vi "Facade.vi"(0 "Data In":T8, 2 "Display State In":T2={"Nspeakers"=0, "actions"=[], "Wspeaker"=13, "hover"={"type"=enum."None", "index"=0}, "locked"=FALSE, "states"=[], "sel speak"=13, "selected"=refnum, "Events"={"Selection change"=refnum}}, 3 "Container State":T7) -> (6 "Data Out":T8, 7 "Display State Out":T2={"Nspeakers"=0, "actions"=[], "Wspeaker"=13, "hover"={"type"=enum."None", "index"=0}, "locked"=FALSE, "states"=[], "sel speak"=13, "selected"=refnum, "Events"={"Selection change"=refnum}}, 8 "Action":T1)   [LabVIEW 2015, in "SAC Config.xctl"]
uses:
  SAC Config.xctl
  <vilib>/_xctls/Action.ctl
  <vilib>/_xctls/XControlSupport.lvlib
  Speaker State.ctl
  Hover Item.ctl
  <vilib>/_xctls/Container State.ctl
  Data.vi
  State.vi
  Hover Data.ctl
  Events.ctl
  Selection changed.ctl
panel:
  out "angle":string
  out "selected":picture
  out "speakers":picture
  out "back":picture
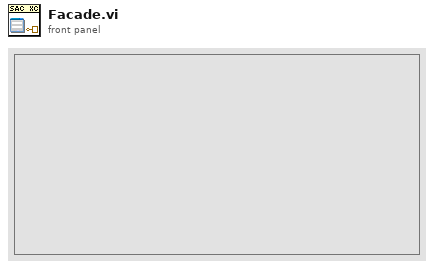
[diagram p1: front panel]
types:
  T1 = typedef "XControlSupport.lvlib/Action.ctl" = cluster{"Data Changed?":bool, "State Changed?":bool, "Action Name":string}
  T2 = typedef "SAC Config.xctl/State.vi" = cluster{"Nspeakers":i32, "actions":string[], "Wspeaker":i32, "hover":T3, "locked":bool, "states":T5[], "sel speak":i32, "selected":refnum<vi>, "Events":T6}
  T3 = typedef "SAC Config.xctl/Hover Data.ctl" = cluster{"type":T4, "index":i32}
  T4 = typedef "SAC Config.xctl/Hover Item.ctl" = enum16{"None", "Speaker"}
  T5 = typedef "SAC Config.xctl/Speaker State.ctl" = cluster{"cal":bool, "selected":bool}
  T6 = typedef "SAC Config.xctl/Events.ctl" = cluster{"Selection change":refnum<user-event>}
  T7 = typedef "XControlSupport.lvlib/Container State.ctl" = cluster{"Indicator?":bool, "Run Mode?":bool, " Refnum":refnum<vi>}
  T8 = typedef "SAC Config.xctl/Data.vi" = i32
  T9 = typedef "LVPoint32TypeDef.ctl" = cluster{"Horizontal":i32, "Vertical":i32}
  T10 = cluster{"Min Control Width":i32, "Min Control Height":i32}
  T11 = typedef "LVPointTypeDef.ctl" = cluster{"Horizontal":i16, "Vertical":i16}
  T12 = typedef "SAC Config.xctl/Layout.ctl" = cluster{"origin":cluster{"X":i32, "Y":i32}, "Items":T13[], "ring diameter":i32}
  T13 = typedef "SAC Config.xctl/Item.ctl" = cluster{"center":cluster{"X":i32, "Y":i32}, "angle":dbl}
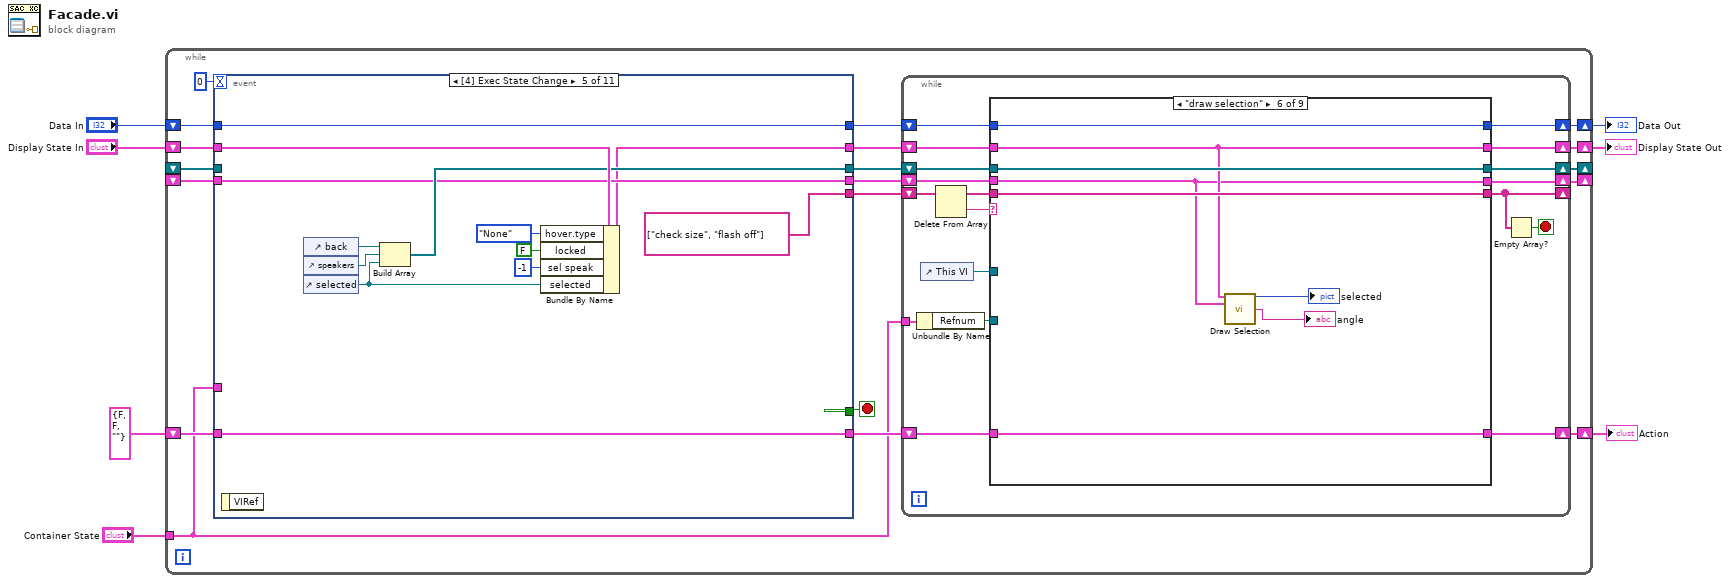
[diagram p0: block diagram]
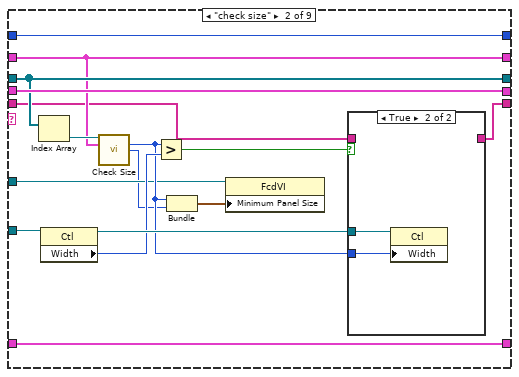
[diagram p3: hidden frame]
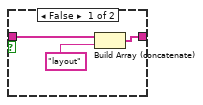
[diagram p4: hidden frame]
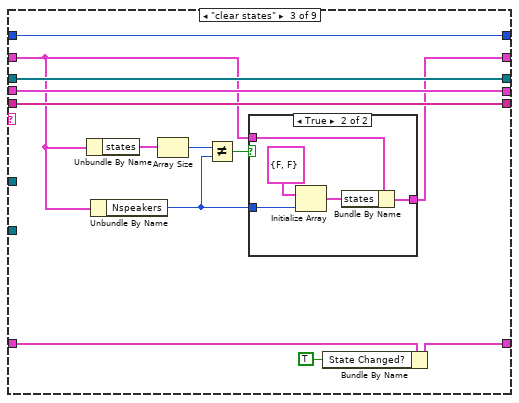
[diagram p5: hidden frame]
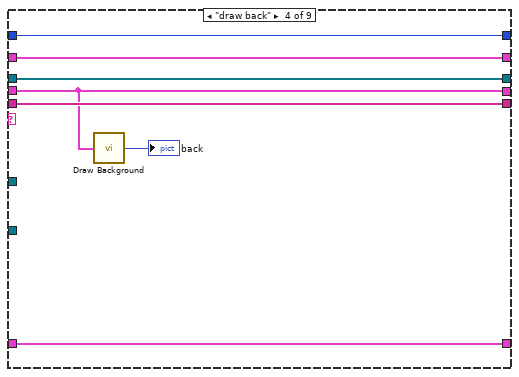
[diagram p7: hidden frame]
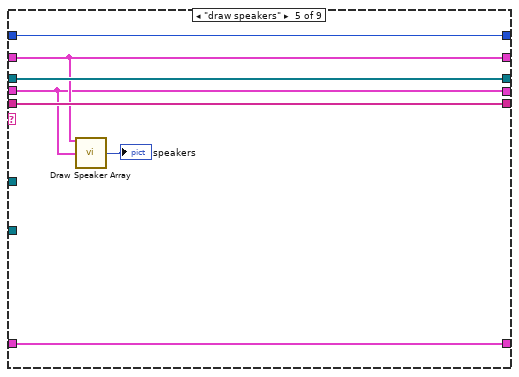
[diagram p8: hidden frame]
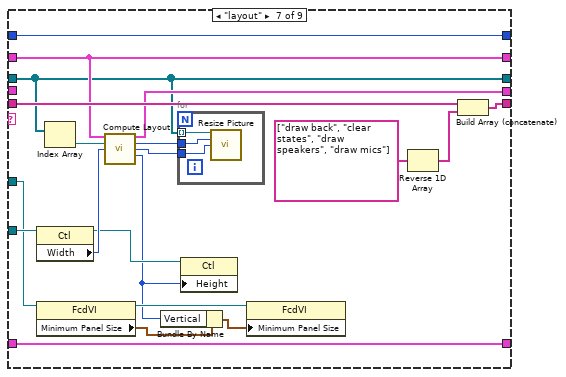
[diagram p9: hidden frame]
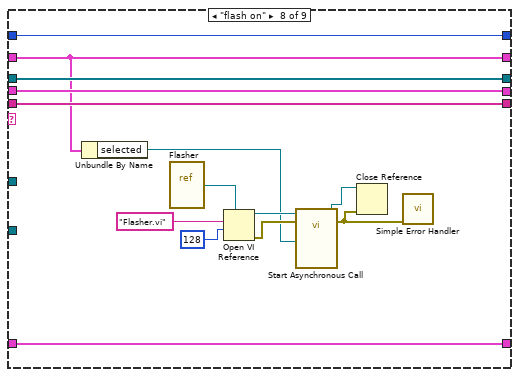
[diagram p10: hidden frame]
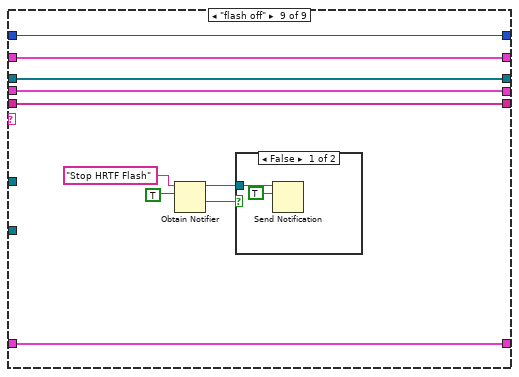
[diagram p11: hidden frame]
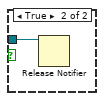
[diagram p12: hidden frame]
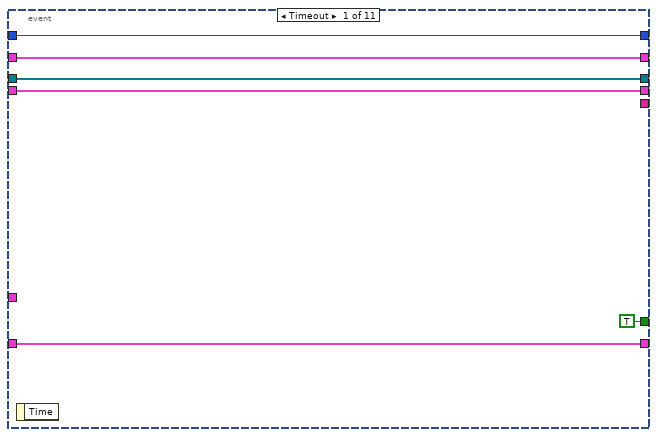
[diagram p13: hidden frame]
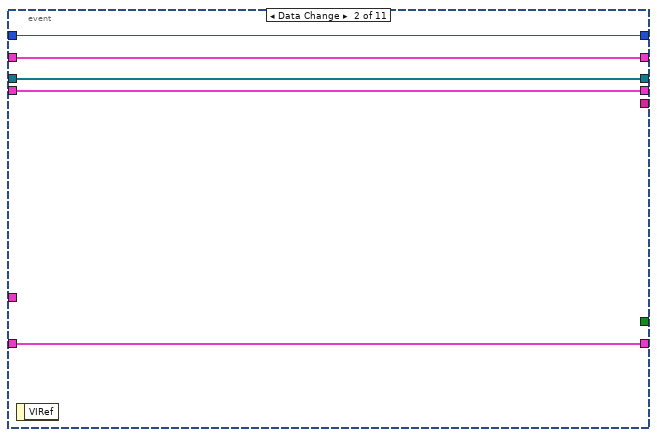
[diagram p14: hidden frame]
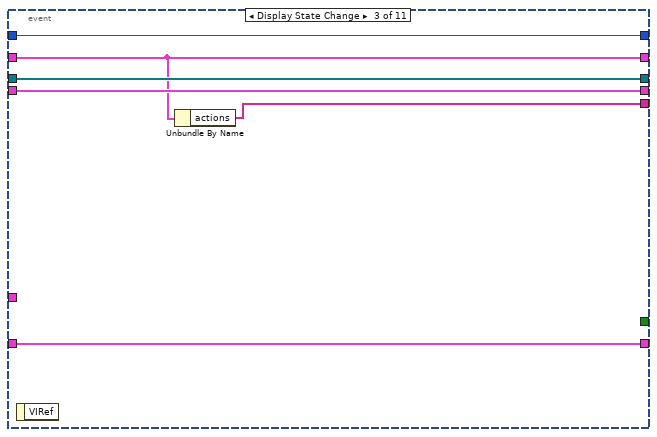
[diagram p15: hidden frame]
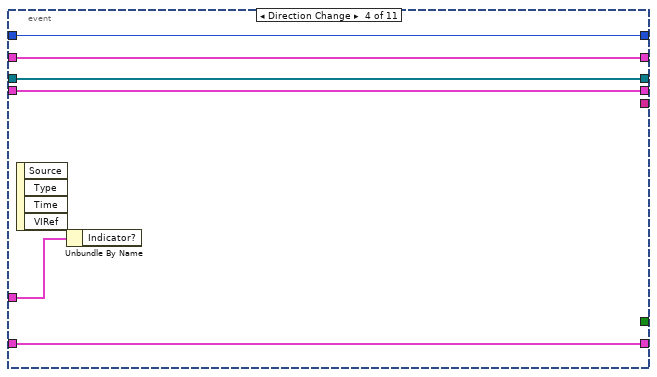
[diagram p16: hidden frame]
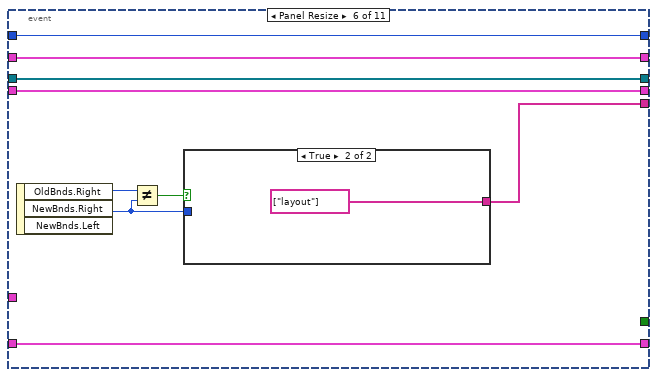
[diagram p17: hidden frame]
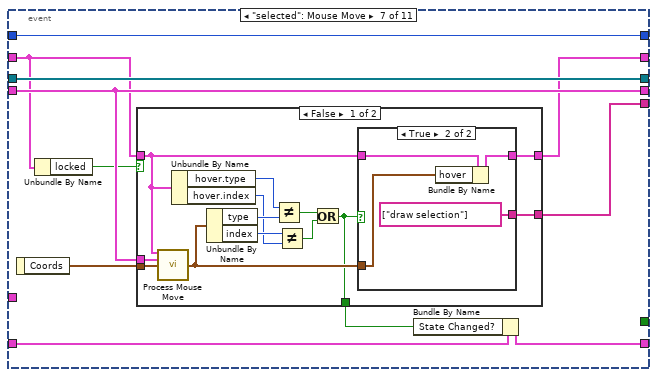
[diagram p19: hidden frame]
diagram:
  n1 = while {
    shift-right: [w15] -> w4
    shift-left: "Display State In" -> [w26]
    tunnel: "Container State" -> [w11]
    shift-right: [w16] -> w7
    shift-left: "Data In" -> [w23]
    shift-right: [w13] -> w2
    shift-left: T1 {"Data Changed?"=FALSE, "State Changed?"=FALSE, "Action Name"=""} ("Action") -> [w22]
    shift-right: [w14] -> _
    shift-left: _ -> [w21]
    shift-right: [w10] -> _
    shift-left: _ -> [w9]
    stop <- w25 stop-if-true
    n2 = event shown="[4] Exec State Change" {
      selector: _ -> [_ _ _ _ _ _ _ _ _ _ _]
      dyn-events: _ -> [_ _ _ _ _ _ _ _ _ _ _]
      timeout: 0 -> [_ _ _ _ _ _ _ _ _ _ _]
      tunnel: w26 -> [w166 w172 w174 w184 w194 w207 w210 w246 w286 w299 w305]
      tunnel: [w166 w172 w174 w184 w190 w207 w214 w245 w285 w299 w310] -> w18
      tunnel: [TRUE _ _ _ _ _ _ _ _ _ _] -> w25
      tunnel: w11 -> [_ _ _ w185 _ _ _ _ _ _ _]
      tunnel: w23 -> [w165 w173 w179 w183 w198 w206 w219 w252 w290 w303 w318]
      tunnel: [w165 w173 w179 w183 w198 w206 w219 w252 w290 w303 w318] -> w17
      tunnel: [w167 w171 w178 w182 w197 w205 w213 w244 w284 w302 w313] -> w12
      tunnel: w22 -> [w167 w171 w178 w182 w197 w205 w218 w251 w289 w302 w317]
      tunnel: [w164 w170 w177 w181 w193 w204 w217 w250 w288 w301 w316] -> w19
      tunnel: w21 -> [w164 w170 w177 w181 _ w204 w217 w250 w288 w301 w316]
      tunnel: [_ _ w175 _ string[] ["check size", "flash off"] w199 w211 w242 w282 _ string[] ["draw selection", "draw speakers"] ("String")] -> w20
      tunnel: w9 -> [w163 w169 w176 w180 w191 w200 w215 w248 w287 w300 w315]
      tunnel: [w163 w169 w176 w180 w191 w200 w215 w248 w287 w300 w315] -> w8
      event Timeout {
        n3 = event-data() -> ()  [unwired: 1 in, 1 out]
      }
      event Data Change {
        n4 = event-data() -> ()  [unwired: 1 in, 1 out]
      }
      event Display State Change {
        n5 = event-data() -> ()  [unwired: 1 in, 1 out]
        n6 = Unbundle By Name(w174) -> ("actions"=w175:string[])
      }
      event Direction Change {
        n7 = event-data() -> ()  [unwired: 1 in, 4 out]
        n8 = Unbundle By Name(w185) -> ()  [unwired: 1 out]
      }
      event Exec State Change {
        n9 = event-data() -> ()  [unwired: 1 in, 1 out]
        n10 = control-ref of="back"() -> (w195:refnum<vi>)
        n11 = control-ref of="speakers"() -> (w196:refnum<vi>)
        n12 = control-ref of="selected"() -> (w186:refnum<vi>)
        n13 = Build Array(w195, w196, w186) -> (w193:refnum<vi>[])
        n14 = Bundle By Name(cluster=w194, "hover.type"=Hover_Item."None", "locked"=FALSE, "sel speak"=-1, "selected"=w186) -> (w190:T2)
      }
      event Panel Resize {
        n15 = event-data() -> ("OldBnds.Right"=w203:i16, "NewBnds.Right"=w202:i16)  [unwired: 1 in, 1 out]
        n16 = Not Equal?(x=w203, y=w202) -> (x != y?=w201:bool)
        n17 = case shown="True" w201 {
          tunnel: w202 -> [_ _]
          tunnel: [_ string[] ["layout"] ("String")] -> w199
          frame False {
          }
          frame True {
          }
        }
      }
      event "selected": Mouse Move {
        n18 = event-data() -> ("Coords"=w216:T9)  [unwired: 1 in]
        n19 = Unbundle By Name(w210) -> ("locked"=w209:bool)
        n20 = case shown="False" w209 {
          tunnel: w216 -> [w232 _]
          tunnel: w215 -> [w231 _]
          tunnel: [w223 w238] -> w214
          tunnel: [w222 _] -> w212
          tunnel: [w221 _] -> w211
          tunnel: w210 -> [w220 w238]
          frame False {
            n21 = call "Process Mouse Move.vi"("State"=w220, "Layout"=w231, "Coords"=w232) -> ("Hover Data"=w224:T3)  [unwired: 12 in]
            n22 = Unbundle By Name(w220) -> ("hover.type"=w229:T4, "hover.index"=w226:i32)
            n23 = Unbundle By Name(w224) -> ("type"=w230:T4, "index"=w227:i32)
            n24 = Not Equal?(x=w229, y=w230) -> (x != y?=w228:bool)
            n25 = Not Equal?(x=w227, y=w226) -> (x != y?=w225:bool)
            n26 = Or(x=w228, y=w225) -> (x .or. y?=w222:bool)
            n27 = case shown="True" w222 {
              tunnel: w224 -> [_ w235]
              tunnel: w220 -> [w233 w237]
              tunnel: [w233 w236] -> w223
              tunnel: [_ string[] ["draw selection"] ("String")] -> w221
              frame False {
              }
              frame True {
                n28 = Bundle By Name(cluster=w237, "hover"=w235) -> (w236:T2)
              }
            }
          }
          frame True {
          }
        }
        n29 = Bundle By Name(cluster=w218, "State Changed?"=w212) -> (w213:T1)
      }
      event "selected": Mouse Down {
        n30 = event-data() -> ("PlatMods.Shift"=w239:bool)  [unwired: 1 in]
        n31 = Unbundle By Name(w246) -> ("hover.type"=w249:T4, "hover.index"=w247:i32, "sel speak"=w240:i32, "locked"=w241:bool)
        n32 = case shown="False" w241 {
          tunnel: w249 -> [w260 _]
          tunnel: w247 -> [w259 _]
          tunnel: w246 -> [w258 w280]
          tunnel: [w257 w280] -> w245
          tunnel: [w256 _] -> w243
          tunnel: [w255 _] -> w242
          tunnel: w240 -> [w254 _]
          tunnel: w239 -> [w253 _]
          frame False {
            n33 = case shown="\"Speaker\"" w260 {
              tunnel: w258 -> [w264 w267]
              tunnel: w259 -> [_ w270]
              tunnel: [w262 w274] -> w257
              tunnel: [TRUE TRUE] -> w256
              tunnel: [_ string[] ["draw selection", "draw speakers"] ("String")] -> w255
              tunnel: w254 -> [_ w273]
              tunnel: w253 -> [_ w272]
              frame "None", Default {
                n34 = Bundle By Name(cluster=w264, "sel speak"=-1) -> (w262:T2)
              }
              frame "Speaker" {
                n35 = Unbundle By Name(w267) -> ("Events.Selection change"=w269:refnum<user-event>)
                n36 = Unbundle By Name(w267) -> ("states"=w276:T5[])
                n37 = call "Update Speaker Selection.vi"("states in"=w276, "index"=w270, "sel speak"=w273, "Shift"=w272) -> ("states out"=w266:T5[])  [unwired: 11 in]
                n38 = Bundle By Name(cluster=w267, "states"=w266, "sel speak"=w270) -> (w274:T2)
                n39 = for {
                  tunnel: w266 -> [w279] mode=indexing
                  tunnel: [w277] -> w265 mode=indexing if=w278
                  i -> [w277]
                  n40 = Unbundle By Name(w279) -> ("selected"=w278:bool)
                }
                n41 = Bundle(w265) -> (w268:cluster{i32[]})  [unwired: 1 in]
                n42 = Generate User Event(user event=w269, event data cluster=w268) -> ()  [unwired: 2 in, 2 out]
              }
            }
          }
          frame True {
          }
        }
        n43 = Bundle By Name(cluster=w251, "State Changed?"=w243) -> (w244:T1)
      }
      event Mouse Leave {
        n44 = event-data() -> ()  [unwired: 1 in, 1 out]
        n45 = Unbundle By Name(w286) -> ("locked"=w281:bool)
        n46 = case shown="False" w281 {
          tunnel: w286 -> [w296 w297]
          tunnel: [w295 w297] -> w285
          tunnel: [TRUE _] -> w283
          tunnel: [string[] ["draw selection"] ("String") _] -> w282
          frame False {
            n47 = Bundle By Name(cluster=w296, "sel speak"=-1, "hover.type"=Hover_Item."None") -> (w295:T2)
          }
          frame True {
          }
        }
        n48 = Bundle By Name(cluster=w289, "State Changed?"=w283) -> (w284:T1)
      }
      event "selected": Shortcut Menu Activation? {
        n49 = event-data() -> ()  [unwired: 1 in, 1 out]
        n50 = Unbundle By Name(w299) -> ("locked"=w298:bool)
        n51 = event-data("Discard?"=w298) -> ()  [unwired: 1 in, 1 out]
      }
      event "selected": Shortcut Menu Selection (User) {
        n52 = event-data() -> ("ItemTag"=w311:string)  [unwired: 1 in]
        n53 = Unbundle By Name(w305) -> ("states"=w314:T5[])
        n54 = for {
          tunnel: w314 -> [w323] mode=indexing
          tunnel: w311 -> [w325]
          tunnel: [w324] -> w309 mode=indexing
          tunnel: [w321] -> w306 mode=indexing if=w320
          i -> [w321]
          n55 = Unbundle By Name(w323) -> ("selected"=w322:bool)
          n56 = Unbundle By Name(w323) -> ("cal"=w319:bool)
          n57 = case shown="\"cmClearAll\"" w325 {
            tunnel: w319 -> [_ _ w329 _ w334]
            tunnel: [FALSE TRUE w328 FALSE w331] -> w320
            tunnel: w322 -> [_ _ _ _ w332]
            frame "False", Default {
            }
            frame "cmSelectAll" {
            }
            frame "cmSelectIncomplete" {
              n58 = Not(x=w329) -> (.not. x?=w328:bool)
            }
            frame "cmClearAll" {
            }
            frame "cmClearComplete" {
              n59 = Not(x=w334) -> (.not. x?=w333:bool)
              n60 = And(x=w333, y=w332) -> (x .and. y?=w331:bool)
            }
          }
          n61 = Bundle By Name(cluster=w323, "selected"=w320) -> (w324:T5)
        }
        n62 = Unbundle By Name(w305) -> ("Events.Selection change"=w304:refnum<user-event>)
        n63 = Bundle By Name(cluster=w317, "State Changed?"=TRUE) -> (w313:T1)
        n64 = Bundle By Name(cluster=w305, "states"=w309) -> (w310:T2)
        n65 = Bundle(w306) -> (w307:cluster{i32[]})  [unwired: 1 in]
        n66 = Generate User Event(user event=w304, event data cluster=w307) -> ()  [unwired: 2 in, 2 out]
      }
    }
    n67 = while {
      shift-right: [w39] -> w16
      shift-left: w17 -> [w43]
      shift-right: [w38] -> w15
      shift-left: w18 -> [w42]
      shift-right: [w37] -> w14
      shift-left: w19 -> [w41]
      shift-right: [w35] -> w13
      shift-left: w12 -> [w40]
      shift-right: [w36] -> _
      shift-left: w20 -> [w34]
      tunnel: w11 -> [w28]
      shift-right: [w30] -> w10
      shift-left: w8 -> [w29]
      stop <- w44 stop-if-true
      n68 = Unbundle By Name(w28) -> ("Refnum"=w27:refnum<vi>)
      n69 = control-ref of="This VI"() -> (w31:refnum<vi>)
      n70 = Delete From Array(array=w34) -> (deleted portion=w32:string, array with subset deleted=w33:string[])  [unwired: 2 in]
      n71 = case shown="\"draw selection\"" w32 {
        tunnel: w43 -> [w50 w66 w84 w97 w104 w112 w132 w149 w159]
        tunnel: w42 -> [w49 w61 w76 w96 w100 w108 w129 w144 w158]
        tunnel: w41 -> [w48 w63 w83 w95 w103 w111 w122 w148 w157]
        tunnel: w33 -> [w47 w56 w82 w94 w102 w110 w131 w147 w156]
        tunnel: w40 -> [w46 w65 w81 w93 w101 w109 w130 w146 w155]
        tunnel: [w50 w66 w84 w97 w104 w112 w132 w149 w159] -> w39
        tunnel: [w49 w61 w79 w96 w100 w108 w129 w144 w158] -> w38
        tunnel: [w48 w63 w83 w95 w103 w111 w122 w148 w157] -> w37
        tunnel: [w47 w55 w82 w94 w102 w110 w127 w147 w156] -> w36
        tunnel: [w46 w65 w78 w93 w101 w109 w130 w146 w155] -> w35
        tunnel: w31 -> [_ w53 _ _ _ _ w118 _ _]
        tunnel: [w45 w64 w80 w92 w99 w107 w125 w145 w154] -> w30
        tunnel: w29 -> [w45 w64 w80 w92 w99 w107 _ w145 w154]
        tunnel: w27 -> [_ w60 _ _ _ _ w128 _ _]
        frame "False", Default {
        }
        frame "check size" {
          n72 = Index Array(array=w63) -> (element=w62:refnum<vi>)  [unwired: 1 in]
          n73 = property class="Ctl"(reference=w60) -> (reference out=w59:refnum<vi>, "Width"=w58:u32)  [unwired: 1 in, 1 out]
          n74 = call "Check Size.vi"("picture ref"=w62, "State"=w61) -> ("Min Control Width"=w54:i32, "Min Control Height"=w51:i32)  [unwired: 12 in]
          n75 = Greater?(x=w54, y=w58) -> (0:w57:bool)
          n76 = Bundle("Min Control Width"=w54, "Min Control Height"=w51) -> (w52:T10)  [unwired: 1 in]
          n77 = property class="FcdVI"(reference=w53, "Minimum Panel Size"=w52) -> ()  [unwired: 1 in, 2 out]
          n78 = case shown="True" w57 {
            tunnel: w59 -> [_ w71]
            tunnel: w54 -> [_ w70]
            tunnel: w56 -> [w69 _]
            tunnel: [w68 _] -> w55
            frame False {
              n79 = Build Array (concatenate)(w69, "layout" ("String")) -> (w68:string[])
            }
            frame True {
              n80 = property class="Ctl"(reference=w71, "Width"=w70) -> ()  [unwired: 1 in, 2 out]
            }
          }
        }
        frame "clear states" {
          n81 = Unbundle By Name(w76) -> ("states"=w75:T5[])
          n82 = Unbundle By Name(w76) -> ("Nspeakers"=w73:i32)
          n83 = Array Size(array=w75) -> (size(s)=w74:i32)
          n84 = Not Equal?(x=w74, y=w73) -> (x != y?=w72:bool)
          n85 = case shown="True" w72 {
            tunnel: w73 -> [_ w90]
            tunnel: [w85 w87] -> w79
            tunnel: w76 -> [w85 w86]
            frame False {
            }
            frame True {
              n86 = Initialize Array(T5 {"cal"=FALSE, "selected"=FALSE} ("Speaker State"), w90) -> (w88:T5[])
              n87 = Bundle By Name(cluster=w86, "states"=w88) -> (w87:T2)
            }
          }
          n88 = Bundle By Name(cluster=w81, "State Changed?"=TRUE) -> (w78:T1)
        }
        frame "draw back" {
          n89 = call "Draw Background.vi"("Layout"=w92) -> ("2D Picture"=→"back":picture)  [unwired: 14 in]
        }
        frame "draw speakers" {
          n90 = call "Draw Speaker Array.vi"("State"=w100, "Layout"=w99) -> ("2D Picture"=→"speakers":picture)  [unwired: 13 in]
        }
        frame "draw selection" {
          n91 = call "Draw Selection.vi"("Display State In"=w108, "Layout"=w107) -> ("empty picture"=→"selected":picture, "String"=→"angle":string)  [unwired: 12 in]
        }
        frame "layout" {
          n92 = property class="Ctl"(reference=w128) -> (reference out=w119:refnum<vi>, "Width"=w124:u32)  [unwired: 1 in, 1 out]
          n93 = property class="FcdVI"(reference=w118) -> (reference out=w117:refnum<vi>, "Minimum Panel Size"=w116:T11)  [unwired: 1 in, 1 out]
          n94 = Index Array(array=w122) -> (element=w123:refnum<vi>)  [unwired: 1 in]
          n95 = call "Compute Layout.vi"("State"=w129, "picture ref"=w123, "Size"=w124) -> ("Layout"=w125:T12, "Wpict"=w121:u32, "Hpict"=w120:u32, "Hcontrol"=w114:u32)  [unwired: 9 in]
          n96 = Bundle By Name(cluster=w116, "Vertical"=w114) -> (w115:T11)
          n97 = for {
            tunnel: w122 -> [w135] mode=indexing
            tunnel: w121 -> [w134]
            tunnel: w120 -> [w133]
            n98 = call "Resize Picture.vi"("Picture ref"=w135, "new width"=w134, "new height"=w133) -> ()  [unwired: 13 in]
          }
          n99 = property class="Ctl"(reference=w119, "Height"=w114) -> ()  [unwired: 1 in, 2 out]
          n100 = property class="FcdVI"(reference=w117, "Minimum Panel Size"=w115) -> ()  [unwired: 1 in, 2 out]
          n101 = Reverse 1D Array(array=string[] ["draw back", "clear states", "draw speakers", "draw mics"]) -> (reversed array=w113:string[])
          n102 = Build Array (concatenate)(w131, w113) -> (w127:string[])
        }
        frame "flash on" {
          n103 = Unbundle By Name(w144) -> ("selected"=w136:refnum<vi>)
          n104 = vi-ref "Flasher.vi"() -> (w141:refnum<vi>)
          n105 = Open VI Reference(type specifier VI Refnum (for type only)=w141, vi path="Flasher.vi", options=128) -> (vi reference=w142:refnum<vi>, error out=w140:errorcluster)  [unwired: 3 in]
          n106 = call-by-ref "Start Asynchronous Call"(reference=w142, error in=w140, "reference"=w136) -> (reference out=w138:refnum<vi>, error out=w139:errorcluster)  [unwired: 15 in]
          n107 = Close Reference(reference=w138, error in (no error)=w139) -> ()  [unwired: 1 out]
          n108 = call <vilib>:"Simple Error Handler.vi"("error in (no error)"=w139) -> ()  [unwired: 4 in, 5 out]
        }
        frame "flash off" {
          n109 = Obtain Notifier(name (unnamed)="Stop HRTF Flash", notification data type=TRUE) -> (notifier out=w150:refnum<notifier>, created new?=w151:bool)  [unwired: 2 in, 1 out]
          n110 = case shown="False" w151 {
            tunnel: w150 -> [w161 w162]
            frame False {
              n111 = Send Notification(notification=TRUE, notifier=w161) -> ()  [unwired: 1 in, 2 out]
            }
            frame True {
              n112 = Release Notifier(notifier=w162) -> ()  [unwired: 2 in, 3 out]
            }
          }
        }
      }
      n113 = Empty Array?(array=w36) -> (empty?=w44:bool)
    }
  }
  "Display State Out" <- w4
  "Data Out" <- w7
  "Action" <- w2
